vi "InitializeTree.vi"(7 "Selected File":path, 8 "error in (no error)":errorcluster, 10 "Panel":refnum<vi>, 11 "TreeControl in":refnum<vi>) -> (0 "error out":errorcluster, 2 "File list":path[][](array[path]))   [LabVIEW 2022 SP3]
panel:
  out "Array":path[](array[path])
  out "array of strings":string[](array[string])
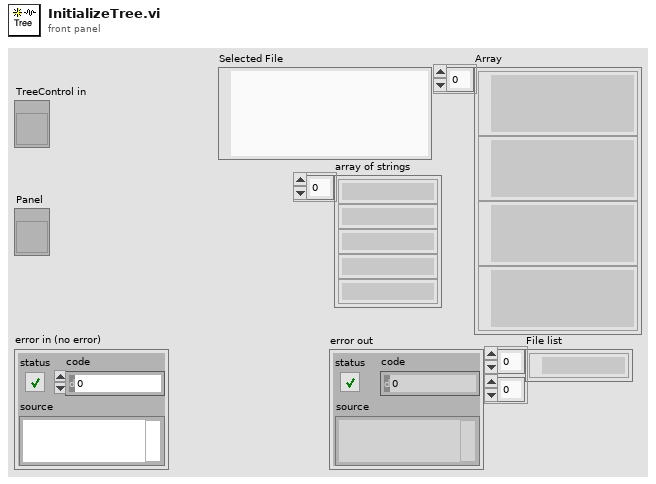
[diagram p1: front panel]
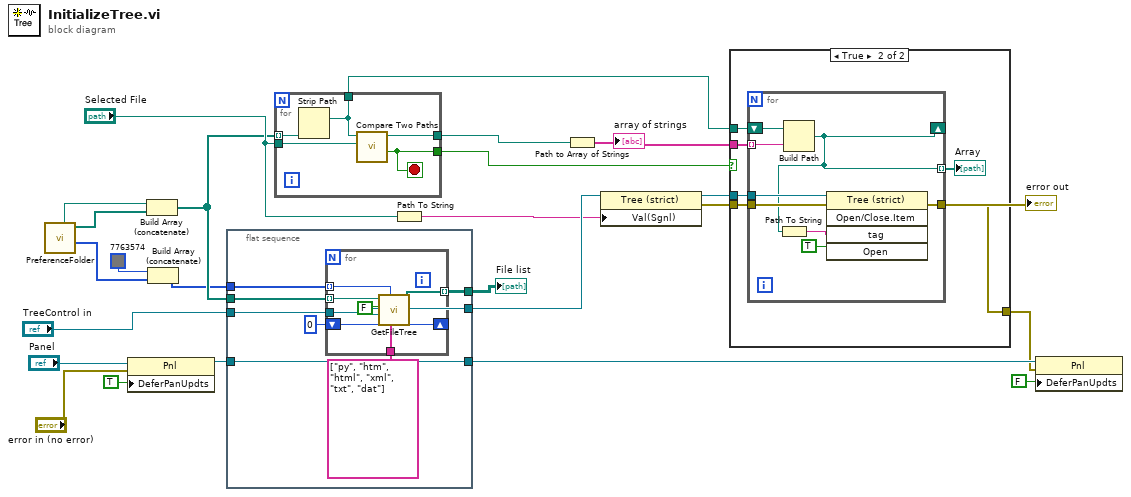
[diagram p0: block diagram]
diagram:
  n1 = call "PreferenceFolder.vi"() -> ("Colors"=w8:u32[], "pythonCodes"=w10:path[], "Examples"=w4:path)  [unwired: 4 in, 5 out]
  n2 = property class="Pnl"(reference="Panel", error in="error in (no error)", "DeferPanUpdts"=TRUE ("Defer Panel Updates")) -> (reference out=w22:refnum<vi>)  [unwired: 1 out]
  n3 = Build Array (concatenate)(w4, w10) -> (w9:path[])
  n4 = Build Array (concatenate)(u32 7763574, w8) -> (w6:u32[])
  n5 = flat-sequence {
    tunnel: w22 -> [w30]
    tunnel: [w30] -> w24
    tunnel: "TreeControl in" -> [w29]
    tunnel: [w29] -> w18
    tunnel: w6 -> [w27]
    tunnel: w9 -> [w26]
    tunnel: [w25] -> w1
    frame #0 {
      n6 = for {
        tunnel: string[] ["py", "htm", "html", "xml", "txt", "dat"] ("patterns") -> [w39]
        tunnel: w29 -> [w37]
        tunnel: w26 -> [w36] mode=indexing
        tunnel: w27 -> [w35] mode=indexing
        shift-right: [w34] -> _
        shift-left: u32 0 ("NumRows") -> [w33]
        tunnel: [w32] -> w25 mode=indexing
        n7 = call "GetFileTree.vi"("patterns"=w39, "Font Color"=w35, "StartRow"=w33, "Tree"=w37, "Open?"=FALSE, "Base Path"=w36) -> ("NumRows"=w34:u32, "File list"=w32:path[])  [unwired: 4 in]
      }
    }
  }
  n8 = for {
    tunnel: w9 -> [w42] mode=indexing
    tunnel: [w41] -> w14
    tunnel: "Selected File" -> [w44]
    tunnel: [w43] -> w12
    tunnel: [w40] -> w11
    stop <- w41 stop-if-true
    n9 = Strip Path(path=w42) -> (stripped path=w40:path)  [unwired: 1 out]
    n10 = call <vilib>:"Compare Two Paths.vi"("Path 2"=w44, "Path 1"=w40) -> ("Path 2 Relative to Path 1?"=w41:bool, "Relative Path from 1 to 2"=w43:path)  [unwired: 6 in, 2 out]
  }
  n11 = Path To String(path="Selected File") -> (string=w3:string)
  n12 = Path to Array of Strings(0:w12) -> (2:w15:string[])  [unwired: 1 out]
  "array of strings" <- w15
  n13 = property class="Tree (strict)"(reference=w18, "Val(Sgnl)"=w3) -> (reference out=w16:refnum<vi>, error out=w5:errorcluster)  [unwired: 1 in]
  "error out" <- w5
  n14 = case shown="True" w14 {
    tunnel: w16 -> [_ w51]
    tunnel: w5 -> [w45 w50]
    tunnel: w11 -> [_ w49]
    tunnel: w15 -> [_ w48]
    tunnel: [w45 w46] -> w2
    frame False {
    }
    frame True {
      n15 = for {
        tunnel: w51 -> [w59]
        tunnel: w50 -> [w58]
        shift-right: [w54] -> _
        shift-left: w49 -> [w56]
        tunnel: w48 -> [w55] mode=indexing
        tunnel: [w54] -> w47 mode=indexing
        tunnel: [w53] -> w46
        n16 = Build Path(base path=w56, name or relative path=w55) -> (appended path=w54:path)
        n17 = Path To String(path=w54) -> (string=w52:string)
        n18 = invoke class="Tree (strict)" method="Open/Close.Item"(reference=w59, error in=w58, "tag"=w52, "Open"=TRUE ("Open?")) -> (error out=w53:errorcluster)  [unwired: 1 in, 4 out]
      }
      "Array" <- w47
    }
  }
  n19 = property class="Pnl"(reference=w24, error in=w2, "DeferPanUpdts"=FALSE ("Defer Panel Updates")) -> ()  [unwired: 2 out]
  "File list" <- w1
